vi "Set Server Address.vi"(8 "error in (no error)":errorcluster, 11 "TwinCAT ADS in":refnum<class "TwinCAT ADS.lvclass">) -> (0 "error out":errorcluster, 3 "TwinCAT ADS out":refnum<class "TwinCAT ADS.lvclass">)   [LabVIEW 2018, in "TwinCAT ADS.lvclass"]
uses:
  TwinCAT ADS.lvclass
  TwinCAT ADS.lvclass/TwinCAT ADS.ctl
  TwinCAT.Ads
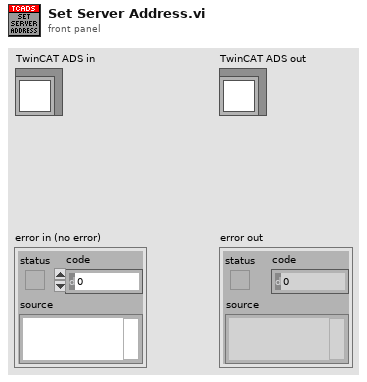
[diagram p1: front panel]
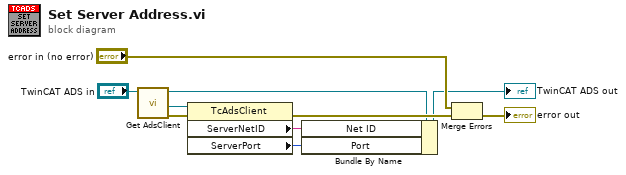
[diagram p0: block diagram]
diagram:
  n1 = call "Get AdsClient.vi"("TwinCAT ADS in"="TwinCAT ADS in") -> ("error out"=w4:errorcluster, ".NET TcAdsClient"=w8:refnum<k24>, "TwinCAT ADS out"=w7:refnum<class "TwinCAT ADS.lvclass">)  [unwired: 8 in]
  n2 = property class="TcAdsClient"(reference=w8, error in=w4) -> (error out=w10:errorcluster, "ServerNetID"=w6:string, "ServerPort"=w5:i32)  [unwired: 1 out]
  n3 = Bundle By Name(cluster=w7, "Net ID"=w6, "Port"=w5) -> (→"TwinCAT ADS out":refnum<class "TwinCAT ADS.lvclass">)
  n4 = Merge Errors("error in (no error)", w10) -> (→"error out":errorcluster)
